vi "xiLIB - LoadFromINI.vi"(6 "IniPath":path, 8 "Error In":errorcluster, 11 "xiCam In":refnum<k24>) -> (0 "Error Out":errorcluster, 3 "xiCam Out":refnum<k24>)   [LabVIEW 2013]
doc: "Dialog based parameter load function."
uses:
  C:/Projects/Cameras3.x/xiLib/xiLIB_64bit/xiLIB/xiCamLib/API/x64/xiApi.NETX64.dll
  xiLIB_64bit/xiLIB/xiCamLib/API/x64/xiApi.NETX64.dll
  xiCam/PRM/PRM/PRM_v2.ctl
  <vilib>/Utility/config.llb/NI_LVConfig.lvlib
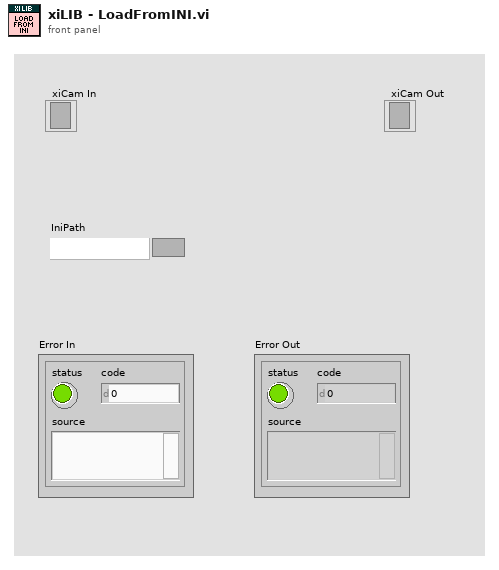
[diagram p1: front panel]
types:
  T1 = typedef "PRM_v2.ctl" = enum16{"ACQ_BUFFER_SIZE", "ACQ_FRAME_BURST_COUNT", "ACQ_TIMING_MODE", "ACQ_TRANSPORT_BUFFER_SIZE", "AE_MAX_LIMIT", "AEAG", "AEAG_LEVEL", "API_VERSION", "AG_MAX_LIMIT", "APPLY_CMS", "AUTO_BANDWIDTH_CALCULATION", "AUTO_WB", "AVAILABLE_BANDWIDTH", "AVAILABLE_BANDWIDTH_MAX", "AVAILABLE_BANDWIDTH_MIN", "BPC", "BUFFER_POLICY", "BUFFERS_QUEUE_SIZE", "CC_MATRIX_00", "CC_MATRIX_01", "CC_MATRIX_02", "CC_MATRIX_03", "CC_MATRIX_10", "CC_MATRIX_11", "CC_MATRIX_12", "CC_MATRIX_13", "CC_MATRIX_20", "CC_MATRIX_21", "CC_MATRIX_22", "CC_MATRIX_23", "CC_MATRIX_30", "CC_MATRIX_31", "CC_MATRIX_32", "CC_MATRIX_33", "CHIP_TEMP", "CMS", "COLOR_FILTER_ARRAY", "COOLING", "DEBOUNCE_EN", "DEBOUNCE_POL", "DEBOUNCE_T0", "DEBOUNCE_T1", "DEBUG_LEVEL", "DEFAULT_CC_MATRIX", "DEVICE_INSTANCE_PATH", "DEVICE_MODEL_ID", "DEVICE_NAME", "DEVICE_SN", "DEVICE_TYPE", "DEVICE_USER_ID", "DOWNSAMPLING", "DOWNSAMPLING_MAX", "DOWNSAMPLING_MIN", "DOWNSAMPLING_TYPE", "DRV_VERSION", "EXP_PRIORITY", "EXPOSURE", "EXPOSURE_DIRECT_UPDATE", "EXPOSURE_MAX", "EXPOSURE_MIN", "FFS_FILE_NAME", "FPGA1_VERSION", "FRAMERATE", "FRAMERATE_MAX", "FRAMERATE_MIN", "FREE_FFS_SIZE", "GAIN", "GAIN_DIRECT_UPDATE", "GAIN_MAX", "GAIN_MIN", "GAMMAC", "GAMMAY", "GPI_LEVEL", "GPI_MODE", "GPI_SELECTOR", "GPI_SELECTOR_MAX", "GPI_SELECTOR_MIN", "GPO_MODE", "GPO_SELECTOR", "GPO_SELECTOR_MAX", "GPO_SELECTOR_MIN", "HDR", "HDR_T1", "HDR_T2", "HEIGHT", "HEIGHT_MAX", "HEIGHT_MIN", "HOUSE_TEMP", "IMAGE_DATA_FORMAT", "IMAGE_IS_COLOR", "INPUT_CMS_PROFILE", "IS_COOLED", "IS_DEVICE_EXIST", "KNEEPOINT1", "KNEEPOINT2", "LED_MODE", "LED_SELECTOR", "LED_SELECTOR_MAX", "LED_SELECTOR_MIN", "LIMIT_BANDWIDTH", "LIMIT_BANDWIDTH_MAX", "LIMIT_BANDWIDTH_MIN", "LUT_EN", "LUT_INDEX", "LUT_INDEX_MAX", "LUT_INDEX_MIN", "LUT_VALUE", "LUT_VALUE_MAX", "LUT_VALUE_MIN", "MANUAL_WB", "MCU1_VERSION", "MCU2_VERSION", "OFFSET_X", "OFFSET_X_MAX", "OFFSET_X_MIN", "OFFSET_Y", "OFFSET_Y_MAX", "OFFSET_Y_MIN", "OUTPUT_CMS_PROFILE", "OUTPUT_DATA_BIT_DEPTH", "OUTPUT_DATA_PACKING", "READ_FILE_FFS", "RECENT_FRAME", "SENSOR_DATA_BIT_DEPTH", "SENSOR_MODE", "SENSOR_TAPS", "SHARPNESS", "SHUTTER_TYPE", "TARGET_TEMP", "TRG_DELAY", "TRG_SELECTOR", "TRG_SOFTWARE", "TRG_SOURCE", "USED_FFS_SIZE", "WB_KB", "WB_KG", "WB_KR", "WIDTH", "WIDTH_MAX", "WIDTH_MIN", "WRITE_FILE_FFS", "ACQ_BUFFER_SIZE_UNIT", "ACQ_TRANSPORT_BUFFER_COMMIT", "AEAG_ROI_HEIGHT", "AEAG_ROI_OFFSET_X", "AEAG_ROU_OFFSET_Y", "AEAG_ROI_WIDTH", "API_CONTEXT_LIST", "BINNING_HORIZONTAL", "BINNING_PATTERN", "BINNING_SELECTOR", "BINNING_VERTICAL", "COLUMN_FPN_CORRECTION", "COUNTER_SELECTOR", "COUNTER_VALUE", "DECIMATION_HORIZONTAL", "DECIMATION_PATTERN", "DECIMATION_SELECTOR", "DECIMATION_VERTICAL", "DEVICE_ID", "DEVICE_LOCATION_PATH", "DEVICE_MANIFEST", "DEVICE_RESET", "DEVICE_SENS_SN", "EXPOSURE_BURST_COUNT", "FFS_ACCESS_KEY", "GAIN_SELECTOR", "HW_REVISION", "IMAGE_BLACK_LEVEL", "IMAGE_DATA_BIT_DEPTH", "IMAGE_DATA_FORMAT_RGB32_ALPHA", "IMAGE_PAYLOAD_SIZE", "LENS_APERTURE_VALUE", "LENS_FEATURE", "LENS_FEATURE_SELECTOR", "LENS_FOCAL_LENGTH", "LENS_FOCUS_DISTANCE", "LENS_FOCUS_MOVE", "LENS_FOCUS_MOVEMENT_VALUE", "LENS_MODE", "OUTPUT_DATA_PACKING_TYPE", "SENSOR_CLOCK_FREQ_HZ", "SENSOR_CLOCK_FREQ_INDEX", "SENSOR_FEATURE_SELECTOR", "SENSOR_FEATURE_VALUE", "SENSOR_OUTPUT_CHANNEL_COUNT", "TRANSPORT_PIXEL_FORMAT", "TS_RST_MODE", "TS_RST_SOURCE"}
  T2 = typedef "NI_LVConfig.lvlib/Config Data RefNum.ctl" = refnum<k1>
  T3 = typedef "xiLIB - PRM_Load_Result.ctl" = enum16{"SUCCESS", "ERROR", "WARNING - Not Valid Parameter", "WARNING - Get Parameter"}
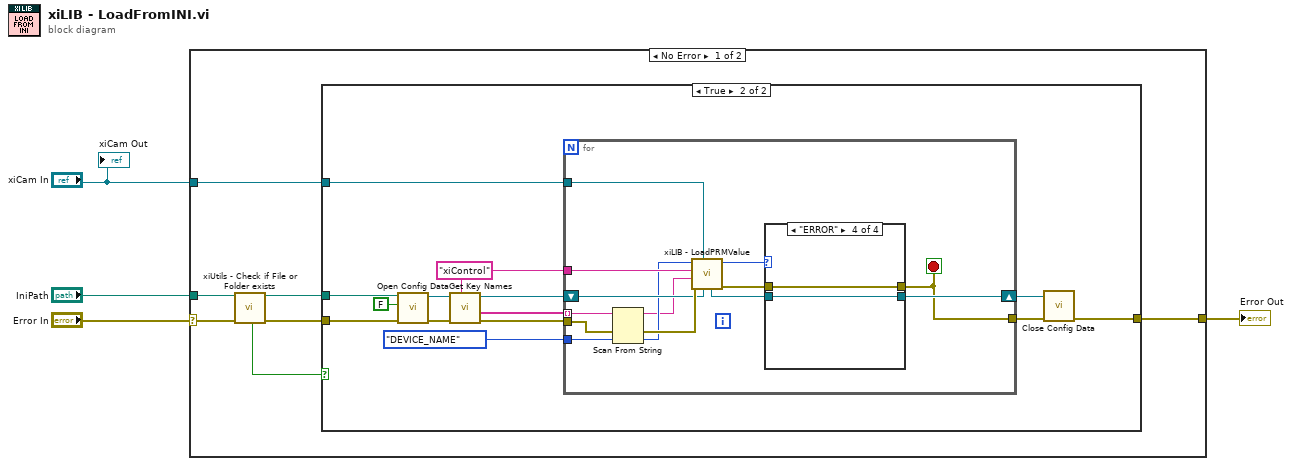
[diagram p0: block diagram]
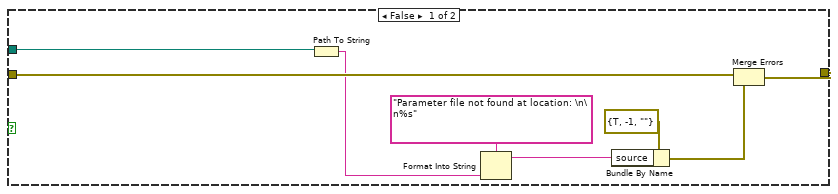
[diagram p2: hidden frame]
diagram:
  n1 = case shown="No Error" "Error In" {
    selector: "Error In" -> [w8 w55]
    tunnel: [w11 w55] -> w3
    tunnel: "IniPath" -> [w9 _]
    tunnel: "xiCam In" -> [w10 _]
    frame No Error {
      n2 = call "xiUtils - Check if File or Folder exists.vi"("error in (no error)"=w8, "path"=w9) -> ("error out"=w7:errorcluster, "file or folder exists?"=w5:bool, "dup path"=w6:path)  [unwired: 7 in]
      n3 = case shown="True" w5 {
        tunnel: [w18 w23] -> w11
        tunnel: w10 -> [_ w26]
        tunnel: w7 -> [w19 w24]
        tunnel: w6 -> [w17 w25]
        frame False {
          n4 = Path To String(path=w17) -> (string=w15:string)
          n5 = Format Into String(format string="Parameter file not found at location: \n\n%s" ("source"), w15) -> (resulting string=w13:string)  [unwired: 2 in, 1 out]
          n6 = Bundle By Name(cluster=errorcluster {"status"=TRUE, "code"=-1, "source"=""} ("error in"), "source"=w13) -> (w12:errorcluster)
          n7 = Merge Errors(w19, w12) -> (w18:errorcluster)
        }
        frame True {
          w31 = "xiControl" ("section")
          n8 = call <vilib>:"Open Config Data.vi"("error in (no error)"=w24, "create file if necessary (T)"=FALSE, "configuration file path"=w25) -> ("error out"=w20:errorcluster, "refnum"=w21:T2)  [unwired: 6 in, 1 out]
          n9 = call <vilib>:"Get Key Names.vi"("section"=w31, "error in (no error)"=w20, "refnum"=w21) -> ("error out"=w28:errorcluster, "key names"=w29:string[], "refnum out"=w33:T2)  [unwired: 5 in, 1 out]
          n10 = for {
            shift-right: [w36] -> w30
            shift-left: w33 -> [w44]
            tunnel: w29 -> [w34] mode=indexing
            tunnel: PRM_v2."DEVICE_NAME" ("PRM") -> [w46]
            tunnel: w28 -> [w43]
            tunnel: w31 -> [w42]
            tunnel: w26 -> [w40]
            tunnel: [w35] -> w27
            stop <- w35 stop-if-true
            n11 = Scan From String(input string=w34, error in=w43, default 1=w46) -> (error out=w45:errorcluster, output 1=w41:T1)  [unwired: 2 in, 2 out]
            n12 = call "xiLIB - LoadPRMValue.vi"("INI Refnum"=w44, "xiCam In"=w40, "error in (no error)"=w45, "key"=w34, "section"=w42, "PRM"=w41) -> ("error out"=w38:errorcluster, "Load_Result"=w39:T3, "INI Refnum out"=w37:T2)  [unwired: 3 in]
            n13 = case shown="\"ERROR\"" w39 {
              tunnel: w38 -> [w47 w49 w51 w53]
              tunnel: w37 -> [w48 w50 w52 w54]
              tunnel: [w48 w50 w52 w54] -> w36
              tunnel: [w47 w49 w51 w53] -> w35
              frame "SUCCESS" {
              }
              frame "WARNING - Not Valid Parameter" {
              }
              frame "WARNING - Get Parameter" {
              }
              frame "ERROR" {
              }
            }
          }
          n14 = call <vilib>:"Close Config Data.vi"("error in (no error)"=w27, "refnum"=w30) -> ("error out"=w23:errorcluster)  [unwired: 8 in, 1 out]
        }
      }
    }
    frame Error {
    }
  }
  "Error Out" <- w3
  "xiCam Out" <- "xiCam In"
